vi "Factorial.vi"(10 "n":u32) -> (2 "n!":ext)   [LabVIEW 2010, in "My Algorithm Library.lvlib"]
uses:
  My Algorithm Library.lvlib
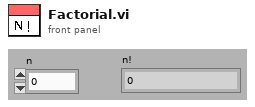
[diagram p1: front panel]
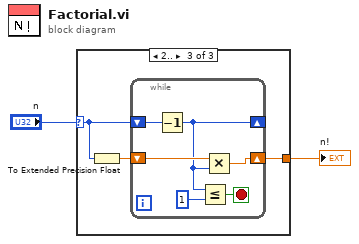
[diagram p0: block diagram]
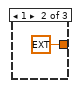
[diagram p3: hidden frame]
diagram:
  n1 = case shown="2.." "n" {
    selector: "n" -> [_ _ w6]
    tunnel: [_ ext 1.0 w4] -> w1
    frame 0, Default {
    }
    frame 1 {
    }
    frame 2.. {
      n2 = To Extended Precision Float(1:w6) -> (0:w5:ext)
      n3 = while {
        shift-right: [w8] -> _
        shift-left: w6 -> [w12]
        shift-right: [w10] -> w4
        shift-left: w5 -> [w11]
        stop <- w9 stop-if-true
        n4 = Decrement(x=w12) -> (x-1=w8:u32)
        n5 = Less Or Equal?(x=w8, y=u32 1) -> (x <= y?=w9:bool)
        n6 = Multiply(x=w11, y=w8) -> (x*y=w10:ext)
      }
    }
  }
  "n!" <- w1
